vi "WLAN_FrameCapture - 2 Channels.vi"(7 "error in (no error)":errorcluster, 9 "Trigger level":dbl format="%0.2f", 10 "session handle":refnum<k15>) -> ()   [LabVIEW 2022 SP3]
uses:
  <instrlib>/niUSRP/niUSRP Fetch Rx Data (2D CDB).vi
  <vilib>/Analysis/NI_AALPro.lvlib
panel:
  out "error out":errorcluster
  out "Waveform Graph":dbl[][](graph)
  out "x <= y?":bool
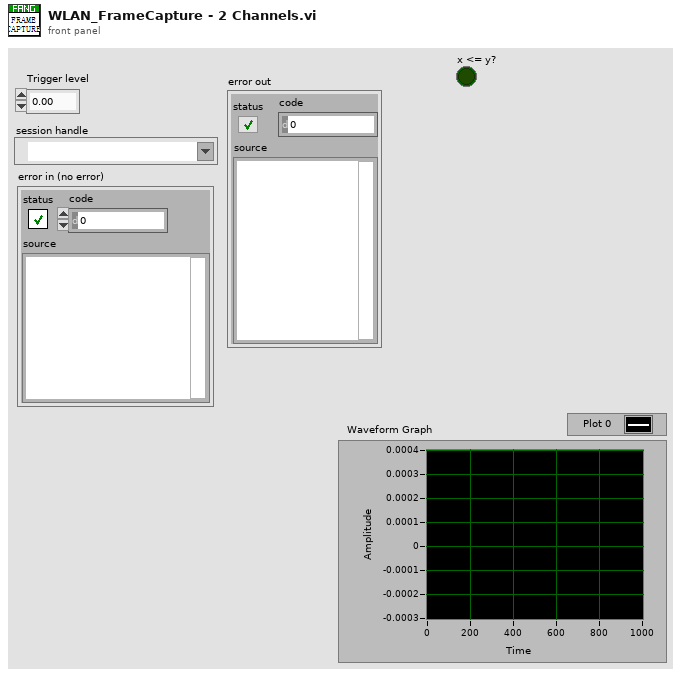
[diagram p1: front panel]
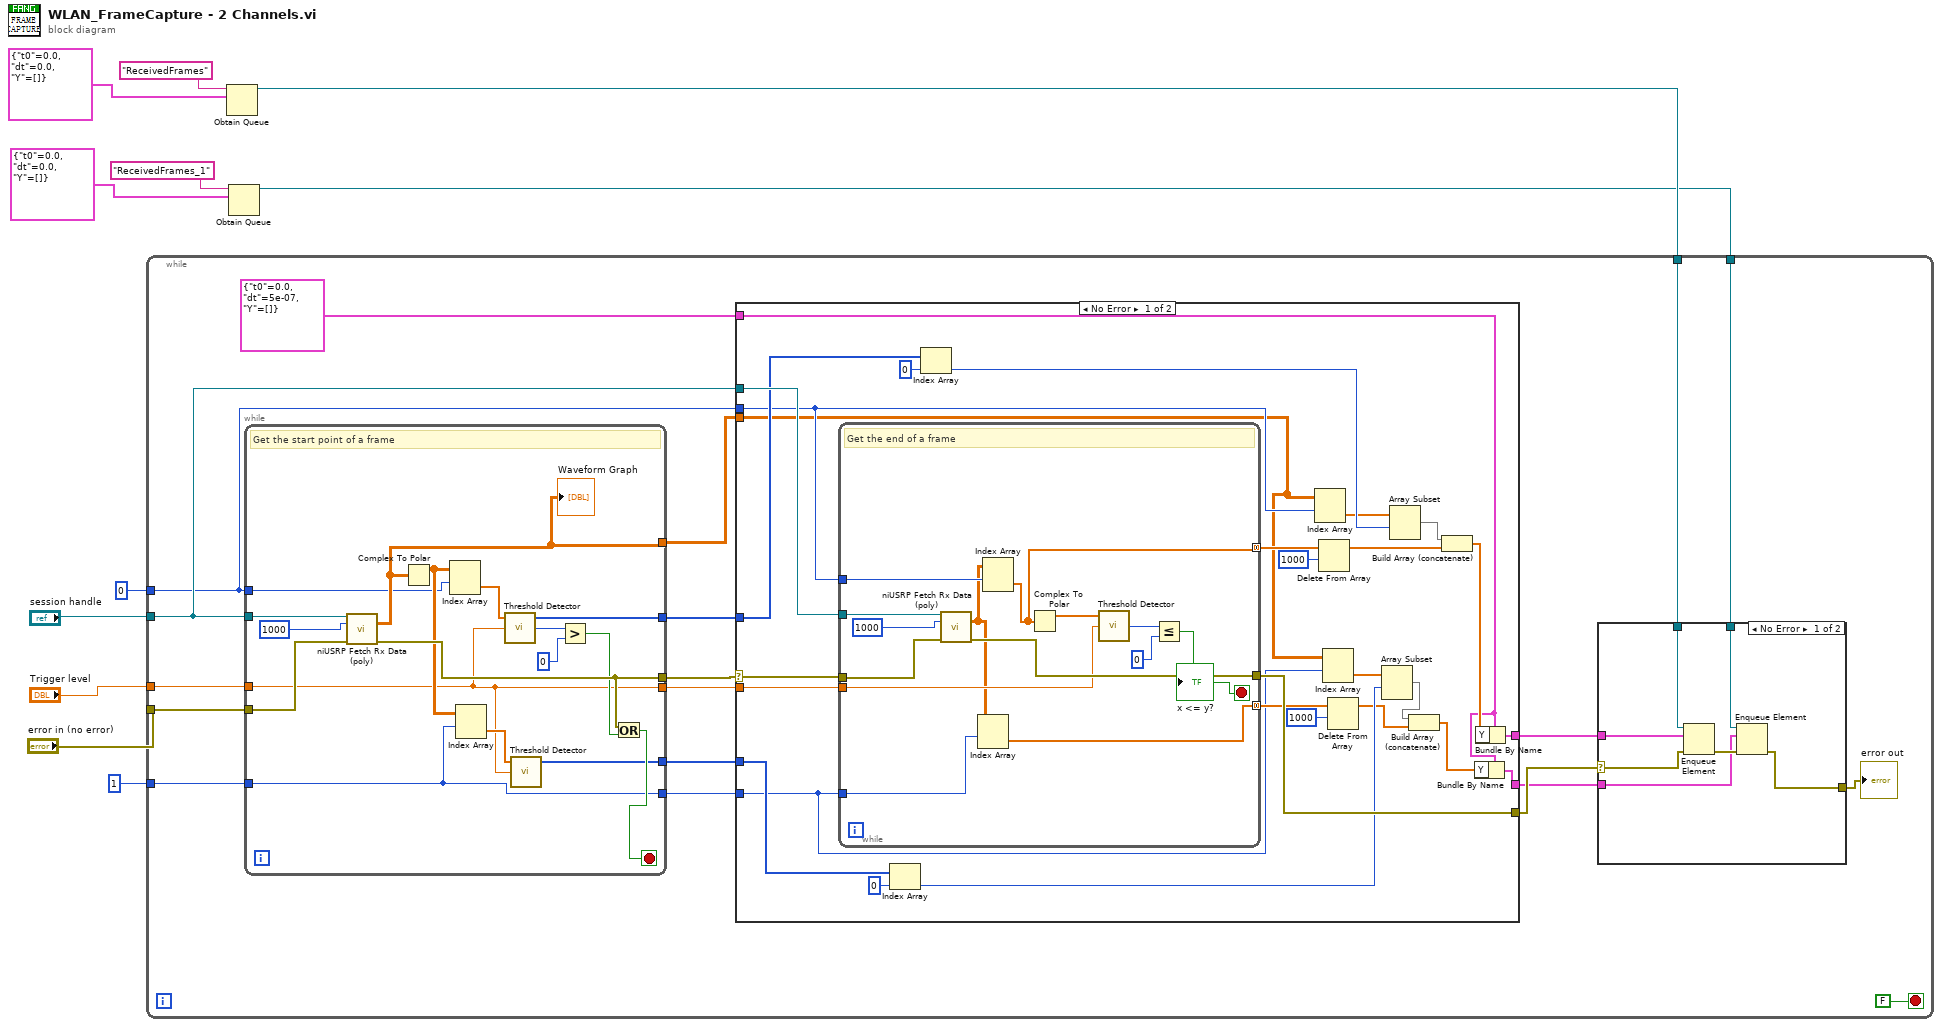
[diagram p0: block diagram]
diagram:
  n1 = Obtain Queue(name (unnamed)="ReceivedFrames", element data type=cluster{"t0":dbl, "dt":dbl, "Y":cdb[]} {"t0"=0.0, "dt"=0.0, "Y"=[]} ("data")) -> (queue out=w6:refnum<queue>)  [unwired: 3 in, 2 out]
  n2 = Obtain Queue(name (unnamed)="ReceivedFrames_1", element data type=cluster{"t0":dbl, "dt":dbl, "Y":cdb[]} {"t0"=0.0, "dt"=0.0, "Y"=[]} ("data")) -> (queue out=w1:refnum<queue>)  [unwired: 3 in, 2 out]
  n3 = while {
    tunnel: "error in (no error)" -> [w30]
    tunnel: "Trigger level" -> [w29]
    tunnel: "session handle" -> [w28]
    tunnel: w6 -> [w24]
    tunnel: 0 -> [w17]
    tunnel: 1 -> [w16]
    tunnel: w1 -> [w12]
    stop <- FALSE stop-if-true
    n4 = while {
      tunnel: w28 -> [w96]
      tunnel: w30 -> [w99]
      tunnel: w29 -> [w85]
      tunnel: [w93] -> w25
      tunnel: [w85] -> w27
      tunnel: [w94] -> w26
      tunnel: [w90] -> w18
      tunnel: w17 -> [w87]
      tunnel: w16 -> [w83]
      tunnel: [w84] -> w15
      tunnel: [w83] -> w14
      stop <- w91 stop-if-true
      # "Get the start point of a frame"
      n5 = call-poly <instrlib>:"niUSRP Fetch Rx Data (poly).vi"("session handle"=w96, "number of samples"=i64 1000, "error in (no error)"=w99) -> ("data"=w90:cdb[][], "error out"=w93:errorcluster)  [unwired: 9 in, 2 out]
      "Waveform Graph" <- w90
      n6 = Complex To Polar(r * e^(i*theta)=w90) -> (r=w88:dbl[][])  [unwired: 1 out]
      n7 = Index Array(array=w88, index (row)=w87) -> (element=w89:dbl[])  [unwired: 1 in]
      n8 = Index Array(array=w88, index (row)=w83) -> (element=w86:dbl[])  [unwired: 1 in]
      n9 = call <vilib>:"Threshold Detector.vi"("threshold"=w85, "X"=w89) -> ("count"=w98:i32, "Indices"=w94:i32[])  [unwired: 1 in, 1 out]
      n10 = call <vilib>:"Threshold Detector.vi"("threshold"=w85, "X"=w86) -> ("Indices"=w84:i32[])  [unwired: 1 in, 2 out]
      n11 = Greater?(x=w98, y=0) -> (0:w92:bool)
      n12 = Or(x=w93, y=w92) -> (x .or. y?=w91:bool)
    }
    n13 = case shown="No Error" w25 {
      selector: w25 -> [w54 w82]
      tunnel: w28 -> [w66 _]
      tunnel: [w65 w82] -> w22
      tunnel: w27 -> [w64 _]
      tunnel: cluster{"t0":dbl, "dt":dbl, "Y":cdb[]} {"t0"=0.0, "dt"=5e-07, "Y"=[]} ("data") -> [w40 w81]
      tunnel: [w63 w81] -> w23
      tunnel: w26 -> [w58 _]
      tunnel: w18 -> [w47 _]
      tunnel: w17 -> [w52 _]
      tunnel: w15 -> [w50 _]
      tunnel: w14 -> [w46 _]
      tunnel: [w39 w81] -> w13
      frame No Error {
        n14 = while {
          tunnel: w66 -> [w78]
          tunnel: [w75] -> w65
          tunnel: w54 -> [w74]
          tunnel: w64 -> [w73]
          tunnel: [w71] -> w62 mode=concatenating
          tunnel: w52 -> [w70]
          tunnel: w46 -> [w68]
          tunnel: [w67] -> w48 mode=concatenating
          stop <- w76 stop-if-true
          # "Get the end of a frame"
          n15 = call-poly <instrlib>:"niUSRP Fetch Rx Data (poly).vi"("session handle"=w78, "number of samples"=i64 1000, "error in (no error)"=w74) -> ("data"=w69:cdb[][], "error out"=w75:errorcluster)  [unwired: 9 in, 2 out]
          n16 = Index Array(array=w69, index (row)=w68) -> (element=w67:cdb[])  [unwired: 1 in]
          n17 = Index Array(array=w69, index (row)=w70) -> (element=w71:cdb[])  [unwired: 1 in]
          n18 = Complex To Polar(r * e^(i*theta)=w71) -> (r=w72:dbl[])  [unwired: 1 out]
          n19 = call <vilib>:"Threshold Detector.vi"("threshold"=w73, "X"=w72) -> ("count"=w80:i32)  [unwired: 1 in, 2 out]
          n20 = Less Or Equal?(x=w80, y=0) -> (x <= y?=w76:bool)
          "x <= y?" <- w76
        }
        n21 = Index Array(array=w50, index=0) -> (element=w44:i32)
        n22 = Index Array(array=w58, index=0) -> (element=w56:i32)
        n23 = Index Array(array=w47, index (row)=w52) -> (element=w53:cdb[])  [unwired: 1 in]
        n24 = Delete From Array(array=w62, length=1000) -> (array with subset deleted=w60:cdb[])  [unwired: 1 in, 1 out]
        n25 = Index Array(array=w47, index (row)=w46) -> (element=w45:cdb[])  [unwired: 1 in]
        n26 = Delete From Array(array=w48, length=1000) -> (array with subset deleted=w42:cdb[])  [unwired: 1 in, 1 out]
        n27 = Array Subset(array=w45, index=w44) -> (w43:cdb[])  [unwired: 1 in]
        n28 = Array Subset(array=w53, index=w56) -> (w55:cdb[])  [unwired: 1 in]
        n29 = Build Array (concatenate)(w43, w42) -> (w41:cdb[])
        n30 = Build Array (concatenate)(w55, w60) -> (w59:cdb[])
        n31 = Bundle By Name(cluster=w40, "Y"=w41) -> (w39:cluster{"t0":dbl, "dt":dbl, "Y":cdb[]})
        n32 = Bundle By Name(cluster=w40, "Y"=w59) -> (w63:cluster{"t0":dbl, "dt":dbl, "Y":cdb[]})
      }
      frame Error {
      }
    }
    n33 = case shown="No Error" w22 {
      selector: w22 -> [w35 w38]
      tunnel: w24 -> [w37 _]
      tunnel: w23 -> [w36 _]
      tunnel: [w33 w38] -> w21
      tunnel: w13 -> [w32 _]
      tunnel: w12 -> [w31 _]
      frame No Error {
        n34 = Enqueue Element(queue=w37, element=w36, error in (no error)=w35) -> (error out=w34:errorcluster)  [unwired: 1 in, 2 out]
        n35 = Enqueue Element(queue=w31, element=w32, error in (no error)=w34) -> (error out=w33:errorcluster)  [unwired: 1 in, 2 out]
      }
      frame Error {
      }
    }
    "error out" <- w21
  }
